vi "serialization tests.vi"() -> ()   [LabVIEW 2014, in "Simple Sequencer TBM tests.lvlib"]
uses:
  <vilib>/NI/TBM Modules/Sequencer/testing/Simple Sequencer TBM tests.lvlib
  <vilib>/NI/TBM Modules/Sequencer/module/configuration/Simple Sequencer TBM configuration.lvclass
panel:
  out "classes equal":bool
  out "no error":errorcluster
  out "no error":errorcluster
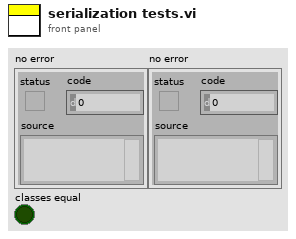
[diagram p1: front panel]
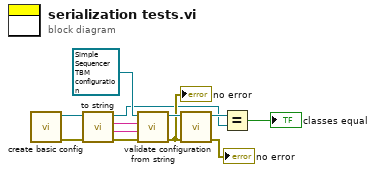
[diagram p0: block diagram]
diagram:
  n1 = call <vilib>:"create basic config.vi"() -> ("error out"=w4:errorcluster, "user tag bus module configuration out"=w3:refnum<class "Simple Sequencer TBM configuration.lvclass">)  [unwired: 8 in, 2 out]
  n2 = call-dynamic "to string.vi"("error in"=w4, "Simple Sequencer TBM configuration in"=w3) -> ("error out"=w12:errorcluster, "data"=w11:string, "version"=w10:string, "Simple Sequencer TBM configuration out"=w1:refnum<class "Simple Sequencer TBM configuration.lvclass">)  [unwired: 6 in]
  n3 = call-dynamic "from string.vi"("error in"=w12, "data"=w11, "version"=w10, "Simple Sequencer TBM configuration in"=refnum<class "Simple Sequencer TBM configuration.lvclass"> refnum ("tag bus configurable plugin module configuration")) -> ("error out"=w7:errorcluster, "Simple Sequencer TBM configuration out"=w9:refnum<class "Simple Sequencer TBM configuration.lvclass">)  [unwired: 6 in]
  "no error" <- w7
  n4 = call-dynamic "validate configuration.vi"("error in"=w7, "Simple Sequencer TBM configuration in"=w9) -> ("error out"=→"no error":errorcluster, "Simple Sequencer TBM configuration out"=w2:refnum<class "Simple Sequencer TBM configuration.lvclass">)  [unwired: 8 in]
  n5 = Equal?(x=w2, y=w1) -> (x = y?=→"classes equal":bool)
